vi "Test Angle.vi"(11 "Test Case In":refnum<class "Vector 2D Tests.lvclass">) -> (0 "error out":errorcluster, 3 "Test Case Out":refnum<class "Vector 2D Tests.lvclass">)   [LabVIEW 2021, in "Vector 2D Tests.lvclass"]
uses:
  Vector 2D Tests.lvclass
  4993e8ee-a06a-463a-9684-69129f64d5ce.vi
  Re-use Libraries/Vector 2D/Vector 2D.lvclass
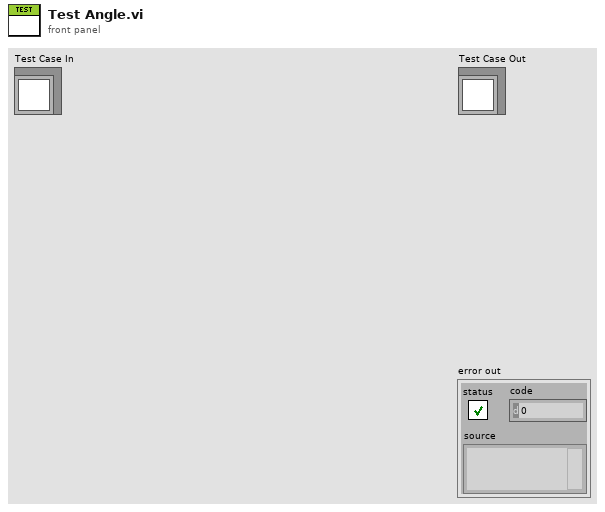
[diagram p1: front panel]
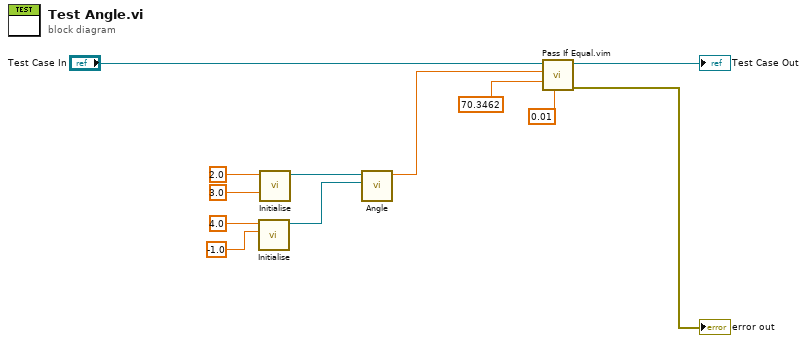
[diagram p0: block diagram]
diagram:
  n1 = call "Initialise.vi"("y"=sgl -1.0 ("x"), "x"=sgl 4.0) -> ("Vector 2D out"=w7:refnum<class "Vector 2D.lvclass">)  [unwired: 9 in]
  n2 = call "Initialise.vi"("y"=sgl 3.0, "x"=sgl 2.0) -> ("Vector 2D out"=w11:refnum<class "Vector 2D.lvclass">)  [unwired: 9 in]
  n3 = call "Angle.vi"("B"=w7, "A"=w11) -> ("Angle [deg]"=w6:dbl)  [unwired: 9 in]
  n4 = call "Pass If Equal.vim"("Delta"=0.01 ("Angle"), "Actual"=70.3462 ("Angle"), "Expected"=w6, "LUnit Test Case In"="Test Case In") -> ("error out"=→"error out":errorcluster, "LUnit Test Case Out"=→"Test Case Out":refnum<class "Vector 2D Tests.lvclass">)  [unwired: 6 in]
